vi "nanocal -- nuclear schottky fit V8.vi"() -> ()   [LabVIEW 2021] (continued)
0.000679567052   ,  \"σητN\" -> 0.003677742744    |>   , \r\"IDS0337_210904_RAW_cal__sam_\" ->   <|    \"ζ\" -> 0.174989526301   ,  \"τ1\" -> 0.032277116931   ,  \"τS\" -> 0.156061636315   ,  \"τN\" -> 0.033861256896   ,  \"τC\" -> 0.001461638306   ,  \"κ0\" -> 0.000000000742   ,  \"mm1\" -> 0.000216209109   ,  \"mm2\" -> 0.025810900049   ,  \"mm3\" -> 0.230869056407   ,  \"T\" -> 0.157000000000   ,  \"B\" -> 5.000000000000   ,  \"θ\" -> 90.000000000000   ,  \"Reoff\" -> -41753012.048192769300   ,  \"Imoff\" -> 0.000000000000   ,  \"στ1\" -> 0.000000000000   ,  \"στS\" -> 0.000000000000   ,  \"στN\" -> 0.000000000000   ,  \"τ11 \" -> 0.000000000000   ,  \"τ12\" -> 0.000000000000   ,  \"τ22\" -> 0.000000000000   ,  \"τN1\" -> 0.000000000000   ,  \"τN2\" -> 0.000000000000   ,  \"σηlogτ1 \" -> 0.000000000000   ,  \"σηlogτS\" -> 0.000000000000   ,  \"σηlogτN\" -> 0.000000000000   ,  \"σlogτ1\" -> 0.000000000000   ,  \"σlogτS\" -> 0.000000000000   ,  \"σlogτN\" -> 0.000000000000   ,  \"σητ1\" -> 0.000000000000   ,  \"σητS \" -> 0.000000000000   ,  \"σητN\" -> 0.000000000000    |>   , \r\"IDS0338_210904_RAW_cal__ref_\" ->   <|    \"ζ\" -> 0.265658527884   ,  \"τ1\" -> 0.023120075726   ,  \"τS\" -> 0.103313442466   ,  \"τN\" -> 0.020697464258   ,  \"τC\" -> 0.000912229768   ,  \"κ0\" -> 0.000000000737   ,  \"mm1\" -> 0.000190421822   ,  \"mm2\" -> 0.018760460104   ,  \"mm3\" -> 0.162036885215   ,  \"T\" -> 0.170000000000   ,  \"B\" -> 5.000000000000   ,  \"θ\" -> 90.000000000000   ,  \"Reoff\" -> 0.000000000000   ,  \"Imoff\" -> 0.000000000000   ,  \"στ1\" -> 0.000288316469   ,  \"στS\" -> 0.000137331811   ,  \"στN\" -> 0.000137381757   ,  \"τ11 \" -> 0.000000000000   ,  \"τ12\" -> 0.000000000000   ,  \"τ22\" -> 0.000000000000   ,  \"τN1\" -> 0.000000000000   ,  \"τN2\" -> 0.000000000000   ,  \"σηlogτ1 \" -> 0.284385432190   ,  \"σηlogτS\" -> 0.006339746651   ,  \"σηlogτN\" -> 0.161800590932   ,  \"σlogτ1\" -> 0.012470394664   ,  \"σlogτS\" -> 0.001329273401   ,  \"σlogτN\" -> 0.006637612960   ,  \"σητ1\" -> 0.006575012728   ,  \"σητS \" -> 0.000654981051   ,  \"σητN\" -> 0.003348861948    |>   , \r\"IDS0338_210904_RAW_cal__sam_\" ->   <|    \"ζ\" -> 0.165649151389   ,  \"τ1\" -> 0.028874600848   ,  \"τS\" -> 0.141983523605   ,  \"τN\" -> 0.021766467668   ,  \"τC\" -> 0.001383503895   ,  \"κ0\" -> 0.000000000838   ,  \"mm1\" -> 0.000195205233   ,  \"mm2\" -> 0.024502619119   ,  \"mm3\" -> 0.196435318758   ,  \"T\" -> 0.170000000000   ,  \"B\" -> 5.000000000000   ,  \"θ\" -> 90.000000000000   ,  \"Reoff\" -> -35397590.361445784600   ,  \"Imoff\" -> 0.000000000000   ,  \"στ1\" -> 0.000000000000   ,  \"στS\" -> 0.000000000000   ,  \"στN\" -> 0.000000000000   ,  \"τ11 \" -> 0.000000000000   ,  \"τ12\" -> 0.000000000000   ,  \"τ22\" -> 0.000000000000   ,  \"τN1\" -> 0.000000000000   ,  \"τN2\" -> 0.000000000000   ,  \"σηlogτ1 \" -> 0.000000000000   ,  \"σηlogτS\" -> 0.000000000000   ,  \"σηlogτN\" -> 0.000000000000   ,  \"σlogτ1\" -> 0.000000000000   ,  \"σlogτS\" -> 0.000000000000   ,  \"σlogτN\" -> 0.000000000000   ,  \"σητ1\" -> 0.000000000000   ,  \"σητS \" -> 0.000000000000   ,  \"σητN\" -> 0.000000000000    |>   , \r\"IDS0339_210904_RAW_cal__ref_\" ->   <|    \"ζ\" -> 0.114039542964   ,  \"τ1\" -> 0.023293546514   ,  \"τS\" -> 0.060135025475   ,  \"τN\" -> 0.005147326644   ,  \"τC\" -> 0.001354301187   ,  \"κ0\" -> 0.000000001349   ,  \"mm1\" -> 0.000136157097   ,  \"mm2\" -> 0.020781344891   ,  \"mm3\" -> 0.076457467431   ,  \"T\" -> 0.255000000000   ,  \"B\" -> 5.000000000000   ,  \"θ\" -> 90.000000000000   ,  \"Reoff\" -> 0.000000000000   ,  \"Imoff\" -> 0.000000000000   ,  \"στ1\" -> 0.000249233332   ,  \"στS\" -> 0.000026082358   ,  \"στN\" -> 0.000027486518   ,  \"τ11 \" -> 0.000000000000   ,  \"τ12\" -> 0.000000000000   ,  \"τ22\" -> 0.000000000000   ,  \"τN1\" -> 0.000000000000   ,  \"τN2\" -> 0.000000000000   ,  \"σηlogτ1 \" -> 0.202736508629   ,  \"σηlogτS\" -> 0.001489466713   ,  \"σηlogτN\" -> 0.146001002326   ,  \"σlogτ1\" -> 0.010699673046   ,  \"σlogτS\" -> 0.000433729889   ,  \"σlogτN\" -> 0.005339959858   ,  \"σητ1\" -> 0.004722452294   ,  \"σητS \" -> 0.000089569119   ,  \"σητN\" -> 0.000751514849    |>   , \r\"IDS0339_210904_RAW_cal__sam_\" ->   <|    \"ζ\" -> 0.070510248751   ,  \"τ1\" -> 0.022152847239   ,  \"τS\" -> 0.078660981887   ,  \"τN\" -> 0.006346817462   ,  \"τC\" -> 0.001852903257   ,  \"κ0\" -> 0.000000001477   ,  \"mm1\" -> 0.000119580835   ,  \"mm2\" -> 0.020081415868   ,  \"mm3\" -> 0.094806474219   ,  \"T\" -> 0.255000000000   ,  \"B\" -> 5.000000000000   ,  \"θ\" -> 90.000000000000   ,  \"Reoff\" -> -9000000.000000000000   ,  \"Imoff\" -> 0.000000000000   ,  \"στ1\" -> 0.000000000000   ,  \"στS\" -> 0.000000000000   ,  \"στN\" -> 0.000000000000   ,  \"τ11 \" -> 0.000000000000   ,  \"τ12\" -> 0.000000000000   ,  \"τ22\" -> 0.000000000000   ,  \"τN1\" -> 0.000000000000   ,  \"τN2\" -> 0.000000000000   ,  \"σηlogτ1 \" -> 0.000000000000   ,  \"σηlogτS\" -> 0.000000000000   ,  \"σηlogτN\" -> 0.000000000000   ,  \"σlogτ1\" -> 0.000000000000   ,  \"σlogτS\" -> 0.000000000000   ,  \"σlogτN\" -> 0.000000000000   ,  \"σητ1\" -> 0.000000000000   ,  \"σητS \" -> 0.000000000000   ,  \"σητN\" -> 0.000000000000    |>   , \r\"IDS0340_210904_RAW_cal__ref_\" ->   <|    \"ζ\" -> 0.076525648542   ,  \"τ1\" -> 0.027695674574   ,  \"τS\" -> 0.050135533571   ,  \"τN\" -> 0.002521537223   ,  \"τC\" -> 0.001686073318   ,  \"κ0\" -> 0.000000001730   ,  \"mm1\" -> 0.000116467999   ,  \"mm2\" -> 0.025407303981   ,  \"mm3\" -> 0.060544663199   ,  \"T\" -> 0.308000000000   ,  \"B\" -> 5.000000000000   ,  \"θ\" -> 90.000000000000   ,  \"Reoff\" -> 0.000000000000   ,  \"Imoff\" -> 0.000000000000   ,  \"στ1\" -> 0.000231753766   ,  \"στS\" -> 0.000008787417   ,  \"στN\" -> 0.000010480438   ,  \"τ11 \" -> 0.000000000000   ,  \"τ12\" -> 0.000000000000   ,  \"τ22\" -> 0.000000000000   ,  \"τN1\" -> 0.000000000000   ,  \"τN2\" -> 0.000000000000   ,  \"σηlogτ1 \" -> 0.162472207290   ,  \"σηlogτS\" -> 0.000540904127   ,  \"σηlogτN\" -> 0.139012219140   ,  \"σlogτ1\" -> 0.008367868614   ,  \"σlogτS\" -> 0.000175273227   ,  \"σlogτN\" -> 0.004156368718   ,  \"σητ1\" -> 0.004499777380   ,  \"σητS \" -> 0.000027118517   ,  \"σητN\" -> 0.000350524485    |>   , \r\"IDS0340_210904_RAW_cal__sam_\" ->   <|    \"ζ\" -> 0.049192434897   ,  \"τ1\" -> 0.021139048522   ,  \"τS\" -> 0.064524263818   ,  \"τN\" -> 0.003413094239   ,  \"τC\" -> 0.002227810965   ,  \"κ0\" -> 0.000000001879   ,  \"mm1\" -> 0.000101271202   ,  \"mm2\" -> 0.019728994700   ,  \"mm3\" -> 0.074815955705   ,  \"T\" -> 0.308000000000   ,  \"B\" -> 5.000000000000   ,  \"θ\" -> 90.000000000000   ,  \"Reoff\" -> -4933734.939759036530   ,  \"Imoff\" -> 0.000000000000   ,  \"στ1\" -> 0.000000000000   ,  \"στS\" -> 0.000000000000   ,  \"στN\" -> 0.000000000000   ,  \"τ11 \" -> 0.000000000000   ,  \"τ12\" -> 0.000000000000   ,  \"τ22\" -> 0.000000000000   ,  \"τN1\" -> 0.000000000000   ,  \"τN2\" -> 0.000000000000   ,  \"σηlogτ1 \" -> 0.000000000000   ,  \"σηlogτS\" -> 0.000000000000   ,  \"σηlogτN\" -> 0.000000000000   ,  \"σlogτ1\" -> 0.000000000000   ,  \"σlogτS\" -> 0.000000000000   ,  \"σlogτN\" -> 0.000000000000   ,  \"σητ1\" -> 0.000000000000   ,  \"σητS \" -> 0.000000000000   ,  \"σητN\" -> 0.000000000000    |>   , \r\"IDS0341_210904_RAW_cal__ref_\" ->   <|    \"ζ\" -> 0.056782811482   ,  \"τ1\" -> 0.026331968848   ,  \"τS\" -> 0.042767805397   ,  \"τN\" -> 0.001889396139   ,  \"τC\" -> 0.002016272015   ,  \"κ0\" -> 0.000000002097   ,  \"mm1\" -> 0.000103939246   ,  \"mm2\" -> 0.024219601276   ,  \"mm3\" -> 0.051217663333   ,  \"T\" -> 0.360000000000   ,  \"B\" -> 5.000000000000   ,  \"θ\" -> 90.000000000000   ,  \"Reoff\" -> 0.000000000000   ,  \"Imoff\" -> 0.000000000000   ,  \"στ1\" -> 0.000101422442   ,  \"στS\" -> 0.000002887305   ,  \"στN\" -> 0.000003653210   ,  \"τ11 \" -> 0.000000000000   ,  \"τ12\" -> 0.000000000000   ,  \"τ22\" -> 0.000000000000   ,  \"τN1\" -> 0.000000000000   ,  \"τN2\" -> 0.000000000000   ,  \"σηlogτ1 \" -> 0.151982642430   ,  \"σηlogτS\" -> 0.000404656843   ,  \"σηlogτN\" -> 0.137111244570   ,  \"σlogτ1\" -> 0.003851684700   ,  \"σlogτS\" -> 0.000067511173   ,  \"σlogτN\" -> 0.001933533055   ,  \"σητ1\" -> 0.004002002206   ,  \"σητS \" -> 0.000017306285   ,  \"σητN\" -> 0.000259057456    |>   , \r\"IDS0341_210904_RAW_cal__sam_\" ->   <|    \"ζ\" -> 0.036062522071   ,  \"τ1\" -> 0.018116162768   ,  \"τS\" -> 0.055032833309   ,  \"τN\" -> 0.002026723445   ,  \"τC\" -> 0.002755523522   ,  \"κ0\" -> 0.000000002282   ,  \"mm1\" -> 0.000091630452   ,  \"mm2\" -> 0.017261892165   ,  \"mm3\" -> 0.062635431951   ,  \"T\" -> 0.360000000000   ,  \"B\" -> 5.000000000000   ,  \"θ\" -> 90.000000000000   ,  \"Reoff\" -> -2587349.397590361540   ,  \"Imoff\" -> 0.000000000000   ,  \"στ1\" -> 0.000000000000   ,  \"στS\" -> 0.000000000000   ,  \"στN\" -> 0.000000000000   ,  \"τ11 \" -> 0.000000000000   ,  \"τ12\" -> 0.000000000000   ,  \"τ22\" -> 0.000000000000   ,  \"τN1\" -> 0.000000000000   ,  \"τN2\" -> 0.000000000000   ,  \"σηlogτ1 \" -> 0.000000000000   ,  \"σηlogτS\" -> 0.000000000000   ,  \"σηlogτN\" -> 0.000000000000   ,  \"σlogτ1\" -> 0.000000000000   ,  \"σlogτS\" -> 0.000000000000   ,  \"σlogτN\" -> 0.000000000000   ,  \"σητ1\" -> 0.000000000000   ,  \"σητS \" -> 0.000000000000   ,  \"σητN\" -> 0.000000000000    |>   , \r\"IDS0342_210904_RAW_cal__ref_\" ->   <|    \"ζ\" -> 0.041076601022   ,  \"τ1\" -> 0.018757031155   ,  \"τS\" -> 0.035968750366   ,  \"τN\" -> 0.001085416882   ,  \"τC\" -> 0.002380872433   ,  \"κ0\" -> 0.000000002638   ,  \"mm1\" -> 0.000088519730   ,  \"mm2\" -> 0.017837018320   ,  \"mm3\" -> 0.041788592031   ,  \"T\" -> 0.438000000000   ,  \"B\" -> 5.000000000000   ,  \"θ\" -> 90.000000000000   ,  \"Reoff\" -> 0.000000000000   ,  \"Imoff\" -> 0.000000000000   ,  \"στ1\" -> 0.000064198355   ,  \"στS\" -> 0.000001597078   ,  \"στN\" -> 0.000001834209   ,  \"τ11 \" -> 0.000000000000   ,  \"τ12\" -> 0.000000000000   ,  \"τ22\" -> 0.000000000000   ,  \"τN1\" -> 0.000000000000   ,  \"τN2\" -> 0.000000000000   ,  \"σηlogτ1 \" -> 0.168171879856   ,  \"σηlogτS\" -> 0.000355670898   ,  \"σηlogτN\" -> 0.139592379603   ,  \"σlogτ1\" -> 0.003422628813   ,  \"σlogτS\" -> 0.000044401831   ,  \"σlogτN\" -> 0.001689865537   ,  \"σητ1\" -> 0.003154405190   ,  \"σητS \" -> 0.000012793038   ,  \"σητN\" -> 0.000151515925    |>   , \r\"IDS0342_210904_RAW_cal__sam_\" ->   <|    \"ζ\" -> 0.027534849374   ,  \"τ1\" -> 0.019066527741   ,  \"τS\" -> 0.046236587360   ,  \"τN\" -> 0.001227722560   ,  \"τC\" -> 0.003332461518   ,  \"κ0\" -> 0.000000002852   ,  \"mm1\" -> 0.000083583563   ,  \"mm2\" -> 0.018352322518   ,  \"mm3\" -> 0.052734315722   ,  \"T\" -> 0.438000000000   ,  \"B\" -> 5.000000000000   ,  \"θ\" -> 90.000000000000   ,  \"Reoff\" -> -1846385.542168676850   ,  \"Imoff\" -> 0.000000000000   ,  \"στ1\" -> 0.000000000000   ,  \"στS\" -> 0.000000000000   ,  \"στN\" -> 0.000000000000   ,  \"τ11 \" -> 0.000000000000   ,  \"τ12\" -> 0.000000000000   ,  \"τ22\" -> 0.000000000000   ,  \"τN1\" -> 0.000000000000   ,  \"τN2\" -> 0.000000000000   ,  \"σηlogτ1 \" -> 0.000000000000   ,  \"σηlogτS\" -> 0.000000000000   ,  \"σηlogτN\" -> 0.000000000000   ,  \"σlogτ1\" -> 0.000000000000   ,  \"σlogτS\" -> 0.000000000000   ,  \"σlogτN\" -> 0.000000000000   ,  \"σητ1\" -> 0.000000000000   ,  \"σητS \" -> 0.000000000000   ,  \"σητN\" -> 0.000000000000    |>   , \r\"IDS0343_210904_RAW_cal__ref_\" ->   <|    \"ζ\" -> 0.030668897536   ,  \"τ1\" -> 0.016422384876   ,  \"τS\" -> 0.030525750501   ,  \"τN\" -> 0.000737103869   ,  \"τC\" -> 0.002827601045   ,  \"κ0\" -> 0.000000003285   ,  \"mm1\" -> 0.000077374536   ,  \"mm2\" -> 0.015772817310   ,  \"mm3\" -> 0.035621445722   ,  \"T\" -> 0.530000000000   ,  \"B\" -> 5.000000000000   ,  \"θ\" -> 90.000000000000   ,  \"Reoff\" -> 0.000000000000   ,  \"Imoff\" -> 0.000000000000   ,  \"στ1\" -> 0.000085303275   ,  \"στS\" -> 0.000001638656   ,  \"στN\" -> 0.000001890230   ,  \"τ11 \" -> 0.000000000000   ,  \"τ12\" -> 0.000000000000   ,  \"τ22\" -> 0.000000000000   ,  \"τN1\" -> 0.000000000000   ,  \"τN2\" -> 0.000000000000   ,  \"σηlogτ1 \" -> 0.166582880232   ,  \"σηlogτS\" -> 0.000279115337   ,  \"σηlogτN\" -> 0.139234460334   ,  \"σlogτ1\" -> 0.005194329317   ,  \"σlogτS\" -> 0.000053681095   ,  \"σlogτN\" -> 0.002564401366   ,  \"σητ1\" -> 0.002735688173   ,  \"σητS \" -> 0.000008520205   ,  \"σητN\" -> 0.000102630259    |>   , \r\"IDS0343_210904_RAW_cal__sam_\" ->   <|    \"ζ\" -> 0.023098882919   ,  \"τ1\" -> 0.017709986922   ,  \"τS\" -> 0.038881575014   ,  \"τN\" -> 0.000747654909   ,  \"τC\" -> 0.003803962289   ,  \"κ0\" -> 0.000000003538   ,  \"mm1\" -> 0.000078528513   ,  \"mm2\" -> 0.017209583260   ,  \"mm3\" -> 0.044770458303   ,  \"T\" -> 0.530000000000   ,  \"B\" -> 5.000000000000   ,  \"θ\" -> 90.000000000000   ,  \"Reoff\" -> -1599397.590361446140   ,  \"Imoff\" -> 0.000000000000   ,  \"στ1\" -> 0.000000000000   ,  \"στS\" -> 0.000000000000   ,  \"στN\" -> 0.000000000000   ,  \"τ11 \" -> 0.000000000000   ,  \"τ12\" -> 0.000000000000   ,  \"τ22\" -> 0.000000000000   ,  \"τN1\" -> 0.000000000000   ,  \"τN2\" -> 0.000000000000   ,  \"σηlogτ1 \" -> 0.000000000000   ,  \"σηlogτS\" -> 0.000000000000   ,  \"σηlogτN\" -> 0.000000000000   ,  \"σlogτ1\" -> 0.000000000000   ,  \"σlogτS\" -> 0.000000000000   ,  \"σlogτN\" -> 0.000000000000   ,  \"σητ1\" -> 0.000000000000   ,  \"σητS \" -> 0.000000000000   ,  \"σητN\" -> 0.000000000000    |>   , \r\"IDS0344_210904_RAW_cal__ref_\" ->   <|    \"ζ\" -> 0.026709812446   ,  \"τ1\" -> 0.026755113102   ,  \"τS\" -> 0.027056221253   ,  \"τN\" -> 0.000433685724   ,  \"τC\" -> 0.002938863970   ,  \"κ0\" -> 0.000000003892   ,  \"mm1\" -> 0.000069295841   ,  \"mm2\" -> 0.024848155483   ,  \"mm3\" -> 0.033000682984   ,  \"T\" -> 0.620000000000   ,  \"B\" -> 5.000000000000   ,  \"θ\" -> 90.000000000000   ,  \"Reoff\" -> 0.000000000000   ,  \"Imoff\" -> 0.000000000000   ,  \"στ1\" -> 0.000318098856   ,  \"στS\" -> 0.000001623783   ,  \"στN\" -> 0.000002850113   ,  \"τ11 \" -> 0.000000000000   ,  \"τ12\" -> 0.000000000000   ,  \"τ22\" -> 0.000000000000   ,  \"τN1\" -> 0.000000000000   ,  \"τN2\" -> 0.000000000000   ,  \"σηlogτ1 \" -> 0.118559715842   ,  \"σηlogτS\" -> 0.000074397800   ,  \"σηlogτN\" -> 0.130425012097   ,  \"σlogτ1\" -> 0.011889273453   ,  \"σlogτS\" -> 0.000060015159   ,  \"σlogτN\" -> 0.006571839401   ,  \"σητ1\" -> 0.003172078607   ,  \"σητS \" -> 0.000002012923   ,  \"σητN\" -> 0.000056563466    |>   , \r\"IDS0344_210904_RAW_cal__sam_\" ->   <|    \"ζ\" -> 0.019239644947   ,  \"τ1\" -> 0.016162010817   ,  \"τS\" -> 0.033688234899   ,  \"τN\" -> 0.000426792406   ,  \"τC\" -> 0.004393456024   ,  \"κ0\" -> 0.000000004224   ,  \"mm1\" -> 0.000073664779   ,  \"mm2\" -> 0.015859557336   ,  \"mm3\" -> 0.039393633044   ,  \"T\" -> 0.620000000000   ,  \"B\" -> 5.000000000000   ,  \"θ\" -> 90.000000000000   ,  \"Reoff\" -> -1105421.686746988450   ,  \"Imoff\" -> 0.000000000000   ,  \"στ1\" -> 0.000000000000   ,  \"στS\" -> 0.000000000000   ,  \"στN\" -> 0.000000000000   ,  \"τ11 \" -> 0.000000000000   ,  \"τ12\" -> 0.000000000000   ,  \"τ22\" -> 0.000000000000   ,  \"τN1\" -> 0.000000000000   ,  \"τN2\" -> 0.000000000000   ,  \"σηlogτ1 \" -> 0.000000000000   ,  \"σηlogτS\" -> 0.000000000000   ,  \"σηlogτN\" -> 0.000000000000   ,  \"σlogτ1\" -> 0.000000000000   ,  \"σlogτS\" -> 0.000000000000   ,  \"σlogτN\" -> 0.000000000000   ,  \"σητ1\" -> 0.000000000000   ,  \"σητS \" -> 0.000000000000   ,  \"σητN\" -> 0.000000000000    |>   , \r\"IDS0346_210904_RAW_cal__ref_\" ->   <|    \"ζ\" -> 0.407818389237   ,  \"τ1\" -> 0.059098367304   ,  \"τS\" -> 0.136395388136   ,  \"τN\" -> 0.197758233370   ,  \"τC\" -> 0.001024329886   ,  \"κ0\" -> 0.000000000393   ,  \"mm1\" -> 0.000295598957   ,  \"mm2\" -> 0.022431935370   ,  \"mm3\" -> 0.507822776049   ,  \"T\" -> 0.122000000000   ,  \"B\" -> 8.000000000000   ,  \"θ\" -> 90.000000000000   ,  \"Reoff\" -> 0.000000000000   ,  \"Imoff\" -> 0.000000000000   ,  \"στ1\" -> 0.000493664169   ,  \"στS\" -> 0.000493598095   ,  \"στN\" -> 0.000812310097   ,  \"τ11 \" -> 0.000000000000   ,  \"τ12\" -> 0.000000000000   ,  \"τ22\" -> 0.000000000000   ,  \"τN1\" -> 0.000000000000   ,  \"τN2\" -> 0.000000000000   ,  \"σηlogτ1 \" -> 0.194694000050   ,  \"σηlogτS\" -> 0.012711324010   ,  \"σηlogτN\" -> 0.173317416285   ,  \"σlogτ1\" -> 0.008353262390   ,  \"σlogτS\" -> 0.003618876720   ,  \"σlogτN\" -> 0.004107591797   ,  \"σητ1\" -> 0.011506097527   ,  \"σητS \" -> 0.001733765972   ,  \"σητN\" -> 0.034274946057    |>   , \r\"IDS0346_210904_RAW_cal__sam_\" ->   <|    \"ζ\" -> 0.199267253863   ,  \"τ1\" -> 0.050205114691   ,  \"τS\" -> 0.125855812683   ,  \"τN\" -> 0.296749666016   ,  \"τC\" -> 0.001624351903   ,  \"κ0\" -> 0.000000000535   ,  \"mm1\" -> 0.000267463038   ,  \"mm2\" -> 0.014047868056   ,  \"mm3\" -> 0.544331047407   ,  \"T\" -> 0.122000000000   ,  \"B\" -> 8.000000000000   ,  \"θ\" -> 90.000000000000   ,  \"Reoff\" -> -35716867.469879508000   ,  \"Imoff\" -> 0.000000000000   ,  \"στ1\" -> 0.000000000000   ,  \"στS\" -> 0.000000000000   ,  \"στN\" -> 0.000000000000   ,  \"τ11 \" -> 0.000000000000   ,  \"τ12\" -> 0.000000000000   ,  \"τ22\" -> 0.000000000000   ,  \"τN1\" -> 0.000000000000   ,  \"τN2\" -> 0.000000000000   ,  \"σηlogτ1 \" -> 0.000000000000   ,  \"σηlogτS\" -> 0.000000000000   ,  \"σηlogτN\" -> 0.000000000000   ,  \"σlogτ1\" -> 0.000000000000   ,  \"σlogτS\" -> 0.000000000000   ,  \"σlogτN\" -> 0.000000000000   ,  \"σητ1\" -> 0.000000000000   ,  \"σητS \" -> 0.000000000000   ,  \"σητN\" -> 0.000000000000    |>   , \r\"IDS0347_210906_RAW_cal__ref_\" ->   <|    \"ζ\" -> 0.290481808635   ,  \"τ1\" -> 0.038323944120   ,  \"τS\" -> 0.067047611498   ,  \"τN\" -> 0.095881318046   ,  \"τC\" -> 0.000911015117   ,  \"κ0\" -> 0.000000000644   ,  \"mm1\" -> 0.000203389328   ,  \"mm2\" -> 0.014222650453   ,  \"mm3\" -> 0.235065739133   ,  \"T\" -> 0.157000000000   ,  \"B\" -> 8.000000000000   ,  \"θ\" -> 90.000000000000   ,  \"Reoff\" -> 0.000000000000   ,  \"Imoff\" -> 0.000000000000   ,  \"στ1\" -> 0.000081642608   ,  \"στS\" -> 0.000055996925   ,  \"στN\" -> 0.000108329720   ,  \"τ11 \" -> 0.000000000000   ,  \"τ12\" -> 0.000000000000   ,  \"τ22\" -> 0.000000000000   ,  \"τN1\" -> 0.000000000000   ,  \"τN2\" -> 0.000000000000   ,  \"σηlogτ1 \" -> 0.166799167293   ,  \"σηlogτS\" -> 0.009320651053   ,  \"σηlogτN\" -> 0.160780135489   ,  \"σlogτ1\" -> 0.002130328947   ,  \"σlogτS\" -> 0.000835181511   ,  \"σlogτN\" -> 0.001129831357   ,  \"σητ1\" -> 0.006392401967   ,  \"σητS \" -> 0.000624927391   ,  \"σητN\" -> 0.015415811306    |>   , \r\"IDS0347_210906_RAW_cal__sam_\" ->   <|    \"ζ\" -> 0.169709128246   ,  \"τ1\" -> 0.042569783210   ,  \"τS\" -> 0.096466158196   ,  \"τN\" -> 0.116379310482   ,  \"τC\" -> 0.001498996005   ,  \"κ0\" -> 0.000000000766   ,  \"mm1\" -> 0.000215022431   ,  \"mm2\" -> 0.017656553883   ,  \"mm3\" -> 0.275164490520   ,  \"T\" -> 0.157000000000   ,  \"B\" -> 8.000000000000   ,  \"θ\" -> 90.000000000000   ,  \"Reoff\" -> -35716867.469879508000   ,  \"Imoff\" -> 0.000000000000   ,  \"στ1\" -> 0.000000000000   ,  \"στS\" -> 0.000000000000   ,  \"στN\" -> 0.000000000000   ,  \"τ11 \" -> 0.000000000000   ,  \"τ12\" -> 0.000000000000   ,  \"τ22\" -> 0.000000000000   ,  \"τN1\" -> 0.000000000000   ,  \"τN2\" -> 0.000000000000   ,  \"σηlogτ1 \" -> 0.000000000000   ,  \"σηlogτS\" -> 0.000000000000   ,  \"σηlogτN\" -> 0.000000000000   ,  \"σlogτ1\" -> 0.000000000000   ,  \"σlogτS\" -> 0.000000000000   ,  \"σlogτN\" -> 0.000000000000   ,  \"σητ1\" -> 0.000000000000   ,  \"σητS \" -> 0.000000000000   ,  \"σητN\" -> 0.000000000000    |>   , \r\"IDS0348_210906_RAW_cal__ref_\" ->   <|    \"ζ\" -> 0.234564712181   ,  \"τ1\" -> 0.031261792512   ,  \"τS\" -> 0.052786157224   ,  \"τN\" -> 0.062944714793   ,  \"τC\" -> 0.000875309632   ,  \"κ0\" -> 0.000000000764   ,  \"mm1\" -> 0.000164501338   ,  \"mm2\" -> 0.012702176672   ,  \"mm3\" -> 0.162147674837   ,  \"T\" -> 0.178000000000   ,  \"B\" -> 8.000000000000   ,  \"θ\" -> 90.000000000000   ,  \"Reoff\" -> 0.000000000000   ,  \"Imoff\" -> 0.000000000000   ,  \"στ1\" -> 0.000050446338   ,  \"στS\" -> 0.000029155358   ,  \"στN\" -> 0.000054402622   ,  \"τ11 \" -> 0.000000000000   ,  \"τ12\" -> 0.000000000000   ,  \"τ22\" -> 0.000000000000   ,  \"τN1\" -> 0.000000000000   ,  \"τN2\" -> 0.000000000000   ,  \"σηlogτ1 \" -> 0.161173739457   ,  \"σηlogτS\" -> 0.007924149958   ,  \"σηlogτN\" -> 0.155365649649   ,  \"σlogτ1\" -> 0.001613673870   ,  \"σlogτS\" -> 0.000552329615   ,  \"σlogτN\" -> 0.000864292135   ,  \"σητ1\" -> 0.005038580001   ,  \"σητS \" -> 0.000418285426   ,  \"σητN\" -> 0.009779446506    |>   , \r\"IDS0348_210906_RAW_cal__sam_\" ->   <|    \"ζ\" -> 0.135783247929   ,  \"τ1\" -> 0.037121050091   ,  \"τS\" -> 0.079201640502   ,  \"τN\" -> 0.079201640502   ,  \"τC\" -> 0.001474311209   ,  \"κ0\" -> 0.000000000894   ,  \"mm1\" -> 0.000173730712   ,  \"mm2\" -> 0.016810842330   ,  \"mm3\" -> 0.201522581240   ,  \"T\" -> 0.178000000000   ,  \"B\" -> 8.000000000000   ,  \"θ\" -> 90.000000000000   ,  \"Reoff\" -> -29680722.891566276600   ,  \"Imoff\" -> 0.000000000000   ,  \"στ1\" -> 0.000000000000   ,  \"στS\" -> 0.000000000000   ,  \"στN\" -> 0.000000000000   ,  \"τ11 \" -> 0.000000000000   ,  \"τ12\" -> 0.000000000000   ,  \"τ22\" -> 0.000000000000   ,  \"τN1\" -> 0.000000000000   ,  \"τN2\" -> 0.000000000000   ,  \"σηlogτ1 \" -> 0.000000000000   ,  \"σηlogτS\" -> 0.000000000000   ,  \"σηlogτN\" -> 0.000000000000   ,  \"σlogτ1\" -> 0.000000000000   ,  \"σlogτS\" -> 0.000000000000   ,  \"σlogτN\" -> 0.000000000000   ,  \"σητ1\" -> 0.000000000000   ,  \"σητS \" -> 0.000000000000   ,  \"σητN\" -> 0.000000000000    |>   , \r\"IDS0349_210906_RAW_cal__ref_\" ->   <|    \"ζ\" -> 0.197057469427   ,  \"τ1\" -> 0.029613620558   ,  \"τS\" -> 0.050911815815   ,  \"τN\" -> 0.036816442025   ,  \"τC\" -> 0.000965034060   ,  \"κ0\" -> 0.000000001032   ,  \"mm1\" -> 0.000156774968   ,  \"mm2\" -> 0.015211417778   ,  \"mm3\" -> 0.120226228199   ,  \"T\" -> 0.200000000000   ,  \"B\" -> 8.000000000000   ,  \"θ\" -> 90.000000000000   ,  \"Reoff\" -> 0.000000000000   ,  \"Imoff\" -> 0.000000000000   ,  \"στ1\" -> 0.000057169127   ,  \"στS\" -> 0.000023609008   ,  \"στN\" -> 0.000037318979   ,  \"τ11 \" -> 0.000000000000   ,  \"τ12\" -> 0.000000000000   ,  \"τ22\" -> 0.000000000000   ,  \"τN1\" -> 0.000000000000   ,  \"τN2\" -> 0.000000000000   ,  \"σηlogτ1 \" -> 0.161376688793   ,  \"σηlogτS\" -> 0.005816962816   ,  \"σηlogτN\" -> 0.148995950079   ,  \"σlogτ1\" -> 0.001930501090   ,  \"σlogτS\" -> 0.000463723546   ,  \"σlogτN\" -> 0.001013649805   ,  \"σητ1\" -> 0.004778948029   ,  \"σητS \" -> 0.000296152139   ,  \"σητN\" -> 0.005485500758    |>   , \r\"IDS0349_210906_RAW_cal__sam_\" ->   <|    \"ζ\" -> 0.113690190882   ,  \"τ1\" -> 0.032691214581   ,  \"τS\" -> 0.068786957350   ,  \"τN\" -> 0.048058332081   ,  \"τC\" -> 0.001613875480   ,  \"κ0\" -> 0.000000001156   ,  \"mm1\" -> 0.000161675745   ,  \"mm2\" -> 0.017372504664   ,  \"mm3\" -> 0.146900362342   ,  \"T\" -> 0.200000000000   ,  \"B\" -> 8.000000000000   ,  \"θ\" -> 90.000000000000   ,  \"Reoff\" -> -14590361.445783138300   ,  \"Imoff\" -> 0.000000000000   ,  \"στ1\" -> 0.000000000000   ,  \"στS\" -> 0.000000000000   ,  \"στN\" -> 0.000000000000   ,  \"τ11 \" -> 0.000000000000   ,  \"τ12\" -> 0.000000000000   ,  \"τ22\" -> 0.000000000000   ,  \"τN1\" -> 0.000000000000   ,  \"τN2\" -> 0.000000000000   ,  \"σηlogτ1 \" -> 0.000000000000   ,  \"σηlogτS\" -> 0.000000000000   ,  \"σηlogτN\" -> 0.000000000000   ,  \"σlogτ1\" -> 0.000000000000   ,  \"σlogτS\" -> 0.000000000000   ,  \"σlogτN\" -> 0.000000000000   ,  \"σητ1\" -> 0.000000000000   ,  \"σητS \" -> 0.000000000000   ,  \"σητN\" -> 0.000000000000    |>   , \r\"IDS0350_210906_RAW_cal__ref_\" ->   <|    \"ζ\" -> 0.116383968065   ,  \"τ1\" -> 0.022837025685   ,  \"τS\" -> 0.041355624864   ,  \"τN\" -> 0.016243225582   ,  \"τC\" -> 0.001144746242   ,  \"κ0\" -> 0.000000001355   ,  \"mm1\" -> 0.000116736213   ,  \"mm2\" -> 0.014664448269   ,  \"mm3\" -> 0.073503020662   ,  \"T\" -> 0.260000000000   ,  \"B\" -> 8.000000000000   ,  \"θ\" -> 90.000000000000   ,  \"Reoff\" -> 0.000000000000   ,  \"Imoff\" -> 0.000000000000   ,  \"στ1\" -> 0.000027906584   ,  \"στS\" -> 0.000007380086   ,  \"στN\" -> 0.000010191855   ,  \"τ11 \" -> 0.000000000000   ,  \"τ12\" -> 0.000000000000   ,  \"τ22\" -> 0.000000000000   ,  \"τN1\" -> 0.000000000000   ,  \"τN2\" -> 0.000000000000   ,  \"σηlogτ1 \" -> 0.162256483080   ,  \"σηlogτS\" -> 0.003668520899   ,  \"σηlogτN\" -> 0.144232966841   ,  \"σlogτ1\" -> 0.001221988557   ,  \"σlogτS\" -> 0.000178454219   ,  \"σlogτN\" -> 0.000627452654   ,  \"σητ1\" -> 0.003705455472   ,  \"σητS \" -> 0.000151713974   ,  \"σητN\" -> 0.002342808617    |>   , \r\"IDS0350_210906_RAW_cal__sam_\" ->   <|    \"ζ\" -> 0.071614468485   ,  \"τ1\" -> 0.024327525692   ,  \"τS\" -> 0.055056024171   ,  \"τN\" -> 0.019709093999   ,  \"τC\" -> 0.001754398678   ,  \"κ0\" -> 0.000000001497   ,  \"mm1\" -> 0.000114067222   ,  \"mm2\" -> 0.016460052715   ,  \"mm3\" -> 0.089627186802   ,  \"T\" -> 0.260000000000   ,  \"B\" -> 8.000000000000   ,  \"θ\" -> 90.000000000000   ,  \"Reoff\" -> -10063253.012048184900   ,  \"Imoff\" -> 0.000000000000   ,  \"στ1\" -> 0.000000000000   ,  \"στS\" -> 0.000000000000   ,  \"στN\" -> 0.000000000000   ,  \"τ11 \" -> 0.000000000000   ,  \"τ12\" -> 0.000000000000   ,  \"τ22\" -> 0.000000000000   ,  \"τN1\" -> 0.000000000000   ,  \"τN2\" -> 0.000000000000   ,  \"σηlogτ1 \" -> 0.000000000000   ,  \"σηlogτS\" -> 0.000000000000   ,  \"σηlogτN\" -> 0.000000000000   ,  \"σlogτ1\" -> 0.000000000000   ,  \"σlogτS\" -> 0.000000000000   ,  \"σlogτN\" -> 0.000000000000   ,  \"σητ1\" -> 0.000000000000   ,  \"σητS \" -> 0.000000000000   ,  \"σητN\" -> 0.000000000000    |>   , \r\"IDS0351_210906_RAW_cal__ref_\" ->   <|    \"ζ\" -> 0.080064937947   ,  \"τ1\" -> 0.017296327437   ,  \"τS\" -> 0.036479707086   ,  \"τN\" -> 0.008116806938   ,  \"τC\" -> 0.001346314476   ,  \"κ0\" -> 0.000000001766   ,  \"mm1\" -> 0.000096730306   ,  \"mm2\" -> 0.013119572667   ,  \"mm3\" -> 0.053593470093   ,  \"T\" -> 0.310000000000   ,  \"B\" -> 8.000000000000   ,  \"θ\" -> 90.000000000000   ,  \"Reoff\" -> 0.000000000000   ,  \"Imoff\" -> 0.000000000000   ,  \"στ1\" -> 0.000031102743   ,  \"στS\" -> 0.000006077841   ,  \"στN\" -> 0.000007305969   ,  \"τ11 \" -> 0.000000000000   ,  \"τ12\" -> 0.000000000000   ,  \"τ22\" -> 0.000000000000   ,  \"τN1\" -> 0.000000000000   ,  \"τN2\" -> 0.000000000000   ,  \"σηlogτ1 \" -> 0.176104217691   ,  \"σηlogτS\" -> 0.002693810692   ,  \"σηlogτN\" -> 0.144358868609   ,  \"σlogτ1\" -> 0.001798228177   ,  \"σlogτS\" -> 0.000166608817   ,  \"σlogτN\" -> 0.000900103833   ,  \"σητ1\" -> 0.003045956212   ,  \"σητS \" -> 0.000098269425   ,  \"σητN\" -> 0.001171733066    |>   , \r\"IDS0351_210906_RAW_cal__sam_\" ->   <|    \"ζ\" -> 0.049866383839   ,  \"τ1\" -> 0.023285662985   ,  \"τS\" -> 0.049370833464   ,  \"τN\" -> 0.009866658615   ,  \"τC\" -> 0.002153040267   ,  \"κ0\" -> 0.000000001928   ,  \"mm1\" -> 0.000098362318   ,  \"mm2\" -> 0.018063601956   ,  \"mm3\" -> 0.069468190575   ,  \"T\" -> 0.310000000000   ,  \"B\" -> 8.000000000000   ,  \"θ\" -> 90.000000000000   ,  \"Reoff\" -> -5536144.578313261270   ,  \"Imoff\" -> 0.000000000000   ,  \"στ1\" -> 0.000000000000   ,  \"στS\" -> 0.000000000000   ,  \"στN\" -> 0.000000000000   ,  \"τ11 \" -> 0.000000000000   ,  \"τ12\" -> 0.000000000000   ,  \"τ22\" -> 0.000000000000   ,  \"τN1\" -> 0.000000000000   ,  \"τN2\" -> 0.000000000000   ,  \"σηlogτ1 \" -> 0.000000000000   ,  \"σηlogτS\" -> 0.000000000000   ,  \"σηlogτN\" -> 0.000000000000   ,  \"σlogτ1\" -> 0.000000000000   ,  \"σlogτS\" -> 0.000000000000   ,  \"σlogτN\" -> 0.000000000000   ,  \"σητ1\" -> 0.000000000000   ,  \"σητS \" -> 0.000000000000   ,  \"σητN\" -> 0.000000000000    |>   , \r\"IDS0352_210906_RAW_cal__ref_\" ->   <|    \"ζ\" -> 0.060178216595   ,  \"τ1\" -> 0.015538327560   ,  \"τS\" -> 0.033922393417   ,  \"τN\" -> 0.005018769313   ,  \"τC\" -> 0.001649636137   ,  \"κ0\" -> 0.000000002110   ,  \"mm1\" -> 0.000089741441   ,  \"mm2\" -> 0.012788298805   ,  \"mm3\" -> 0.045594495906   ,  \"T\" -> 0.360000000000   ,  \"B\" -> 8.000000000000   ,  \"θ\" -> 90.000000000000   ,  \"Reoff\" -> 0.000000000000   ,  \"Imoff\" -> 0.000000000000   ,  \"στ1\" -> 0.000024762200   ,  \"στS\" -> 0.000003463726   ,  \"στN\" -> 0.000003978144   ,  \"τ11 \" -> 0.000000000000   ,  \"τ12\" -> 0.000000000000   ,  \"τ22\" -> 0.000000000000   ,  \"τN1\" -> 0.000000000000   ,  \"τN2\" -> 0.000000000000   ,  \"σηlogτ1 \" -> 0.179978131634   ,  \"σηlogτS\" -> 0.001942969644   ,  \"σηlogτN\" -> 0.143630935441   ,  \"σlogτ1\" -> 0.001593620678   ,  \"σlogτS\" -> 0.000102107372   ,  \"σlogτN\" -> 0.000792653332   ,  \"σητ1\" -> 0.002796559163   ,  \"σητS \" -> 0.000065910181   ,  \"σητN\" -> 0.000720850531    |>   , \r\"IDS0352_210906_RAW_cal__sam_\" ->   <|    \"ζ\" -> 0.036116393265   ,  \"τ1\" -> 0.020310974732   ,  \"τS\" -> 0.044594628397   ,  \"τN\" -> 0.005932938101   ,  \"τC\" -> 0.002747123875   ,  \"κ0\" -> 0.000000002292   ,  \"mm1\" -> 0.000090548575   ,  \"mm2\" -> 0.017024776182   ,  \"mm3\" -> 0.058295213810   ,  \"T\" -> 0.360000000000   ,  \"B\" -> 8.000000000000   ,  \"θ\" -> 90.000000000000   ,  \"Reoff\" -> -2518072.289156645540   ,  \"Imoff\" -> 0.000000000000   ,  \"στ1\" -> 0.000000000000   ,  \"στS\" -> 0.000000000000   ,  \"στN\" -> 0.000000000000   ,  \"τ11 \" -> 0.000000000000   ,  \"τ12\" -> 0.000000000000   ,  \"τ22\" -> 0.000000000000   ,  \"τN1\" -> 0.000000000000   ,  \"τN2\" -> 0.000000000000   ,  \"σηlogτ1 \" -> 0.000000000000   ,  \"σηlogτS\" -> 0.000000000000   ,  \"σηlogτN\" -> 0.000000000000   ,  \"σlogτ1\" -> 0.000000000000   ,  \"σlogτS\" -> 0.000000000000   ,  \"σlogτN\" -> 0.000000000000   ,  \"σητ1\" -> 0.000000000000   ,  \"σητS \" -> 0.000000000000   ,  \"σητN\" -> 0.000000000000    |>   , \r\"IDS0353_210906_RAW_cal__ref_\" ->   <|    \"ζ\" -> 0.043805011586   ,  \"τ1\" -> 0.015641832651   ,  \"τS\" -> 0.031297289619   ,  \"τN\" -> 0.002720036846   ,  \"τC\" -> 0.001830581120   ,  \"κ0\" -> 0.000000002632   ,  \"mm1\" -> 0.000072899501   ,  \"mm2\" -> 0.013753455925   ,  \"mm3\" -> 0.039153514190   ,  \"T\" -> 0.438000000000   ,  \"B\" -> 8.000000000000   ,  \"θ\" -> 90.000000000000   ,  \"Reoff\" -> 0.000000000000   ,  \"Imoff\" -> 0.000000000000   ,  \"στ1\" -> 0.000029789904   ,  \"στS\" -> 0.000002213568   ,  \"στN\" -> 0.000002569992   ,  \"τ11 \" -> 0.000000000000   ,  \"τ12\" -> 0.000000000000   ,  \"τ22\" -> 0.000000000000   ,  \"τN1\" -> 0.000000000000   ,  \"τN2\" -> 0.000000000000   ,  \"σηlogτ1 \" -> 0.171230545078   ,  \"σηlogτS\" -> 0.001043214583   ,  \"σηlogτN\" -> 0.141039696626   ,  \"σlogτ1\" -> 0.001904502144   ,  \"σlogτS\" -> 0.000070727156   ,  \"σlogτN\" -> 0.000944837375   ,  \"σητ1\" -> 0.002678359531   ,  \"σητS \" -> 0.000032649789   ,  \"σητN\" -> 0.000383633172    |>   , \r\"IDS0353_210906_RAW_cal__sam_\" ->   <|    \"ζ\" -> 0.028235631162   ,  \"τ1\" -> 0.018033623612   ,  \"τS\" -> 0.040112967891   ,  \"τN\" -> 0.003332308168   ,  \"τC\" -> 0.002994357278   ,  \"κ0\" -> 0.000000002859   ,  \"mm1\" -> 0.000076791949   ,  \"mm2\" -> 0.016073609718   ,  \"mm3\" -> 0.049549560072   ,  \"T\" -> 0.438000000000   ,  \"B\" -> 8.000000000000   ,  \"θ\" -> 90.000000000000   ,  \"Reoff\" -> -2200000.000000000000   ,  \"Imoff\" -> 0.000000000000   ,  \"στ1\" -> 0.000000000000   ,  \"στS\" -> 0.000000000000   ,  \"στN\" -> 0.000000000000   ,  \"τ11 \" -> 0.000000000000   ,  \"τ12\" -> 0.000000000000   ,  \"τ22\" -> 0.000000000000   ,  \"τN1\" -> 0.000000000000   ,  \"τN2\" -> 0.000000000000   ,  \"σηlogτ1 \" -> 0.000000000000   ,  \"σηlogτS\" -> 0.000000000000   ,  \"σηlogτN\" -> 0.000000000000   ,  \"σlogτ1\" -> 0.000000000000   ,  \"σlogτS\" -> 0.000000000000   ,  \"σlogτN\" -> 0.000000000000   ,  \"σητ1\" -> 0.000000000000   ,  \"σητS \" -> 0.000000000000   ,  \"σητN\" -> 0.000000000000    |>   , \r\"IDS0354_210906_RAW_cal__ref_\" ->   <|    \"ζ\" -> 0.034407438278   ,  \"τ1\" -> 0.012759993552   ,  \"τS\" -> 0.028549472180   ,  \"τN\" -> 0.001373973335   ,  \"τC\" -> 0.002126234468   ,  \"κ0\" -> 0.000000003285   ,  \"mm1\" -> 0.000066111743   ,  \"mm2\" -> 0.011901304001   ,  \"mm3\" -> 0.033871846896   ,  \"T\" -> 0.530000000000   ,  \"B\" -> 8.000000000000   ,  \"θ\" -> 90.000000000000   ,  \"Reoff\" -> 0.000000000000   ,  \"Imoff\" -> 0.000000000000   ,  \"στ1\" -> 0.000105401331   ,  \"στS\" -> 0.000005152140   ,  \"στN\" -> 0.000005607099   ,  \"τ11 \" -> 0.000000000000   ,  \"τ12\" -> 0.000000000000   ,  \"τ22\" -> 0.000000000000   ,  \"τN1\" -> 0.000000000000   ,  \"τN2\" -> 0.000000000000   ,  \"σηlogτ1 \" -> 0.184333164792   ,  \"σηlogτS\" -> 0.000694064017   ,  \"σηlogτN\" -> 0.142381877257   ,  \"σlogτ1\" -> 0.008260296568   ,  \"σlogτS\" -> 0.000180463565   ,  \"σlogτN\" -> 0.004080937594   ,  \"σητ1\" -> 0.002352089994   ,  \"σητS \" -> 0.000019815161   ,  \"σητN\" -> 0.000195628903    |>   , \r\"IDS0354_210906_RAW_cal__sam_\" ->   <|    \"ζ\" -> 0.022962333090   ,  \"τ1\" -> 0.020865157142   ,  \"τS\" -> 0.035948400917   ,  \"τN\" -> 0.001990138096   ,  \"τC\" -> 0.003574397791   ,  \"κ0\" -> 0.000000003542   ,  \"mm1\" -> 0.000073258085   ,  \"mm2\" -> 0.019040364220   ,  \"mm3\" -> 0.044135629011   ,  \"T\" -> 0.530000000000   ,  \"B\" -> 8.000000000000   ,  \"θ\" -> 90.000000000000   ,  \"Reoff\" -> -1700000.000000000000   ,  \"Imoff\" -> 0.000000000000   ,  \"στ1\" -> 0.000000000000   ,  \"στS\" -> 0.000000000000   ,  \"στN\" -> 0.000000000000   ,  \"τ11 \" -> 0.000000000000   ,  \"τ12\" -> 0.000000000000   ,  \"τ22\" -> 0.000000000000   ,  \"τN1\" -> 0.000000000000   ,  \"τN2\" -> 0.000000000000   ,  \"σηlogτ1 \" -> 0.000000000000   ,  \"σηlogτS\" -> 0.000000000000   ,  \"σηlogτN\" -> 0.000000000000   ,  \"σlogτ1\" -> 0.000000000000   ,  \"σlogτS\" -> 0.000000000000   ,  \"σlogτN\" -> 0.000000000000   ,  \"σητ1\" -> 0.000000000000   ,  \"σητS \" -> 0.000000000000   ,  \"σητN\" -> 0.000000000000    |>   , \r\"IDS0355_210906_RAW_cal__ref_\" ->   <|    \"ζ\" -> 0.020775547522   ,  \"τ1\" -> 0.014245155504   ,  \"τS\" -> 0.021871141548   ,  \"τN\" -> 0.000446024292   ,  \"τC\" -> 0.003241636501   ,  \"κ0\" -> 0.000000005421   ,  \"mm1\" -> 0.000057740843   ,  \"mm2\" -> 0.013715964925   ,  \"mm3\" -> 0.026493903416   ,  \"T\" -> 0.830000000000   ,  \"B\" -> 8.000000000000   ,  \"θ\" -> 90.000000000000   ,  \"Reoff\" -> 0.000000000000   ,  \"Imoff\" -> 0.000000000000   ,  \"στ1\" -> 0.000172291727   ,  \"στS\" -> 0.000002161761   ,  \"στN\" -> 0.000002696691   ,  \"τ11 \" -> 0.000000000000   ,  \"τ12\" -> 0.000000000000   ,  \"τ22\" -> 0.000000000000   ,  \"τN1\" -> 0.000000000000   ,  \"τN2\" -> 0.000000000000   ,  \"σηlogτ1 \" -> 0.152304599872   ,  \"σηlogτS\" -> 0.000189712528   ,  \"σηlogτN\" -> 0.136839329472   ,  \"σlogτ1\" -> 0.012094759326   ,  \"σlogτS\" -> 0.000098840802   ,  \"σlogτN\" -> 0.006046063343   ,  \"σητ1\" -> 0.002169602709   ,  \"σητS \" -> 0.000004149230   ,  \"σητN\" -> 0.000061033665    |>   , \r\"IDS0355_210906_RAW_cal__sam_\" ->   <|    \"ζ\" -> 0.015987398390   ,  \"τ1\" -> 0.023974349678   ,  \"τS\" -> 0.025824294014   ,  \"τN\" -> 0.000573136357   ,  \"τC\" -> 0.005688548480   ,  \"κ0\" -> 0.000000005865   ,  \"mm1\" -> 0.000073733721   ,  \"mm2\" -> 0.022561297233   ,  \"mm3\" -> 0.033847323811   ,  \"T\" -> 0.830000000000   ,  \"B\" -> 8.000000000000   ,  \"θ\" -> 90.000000000000   ,  \"Reoff\" -> -599999.999999999999   ,  \"Imoff\" -> 0.000000000000   ,  \"στ1\" -> 0.000000000000   ,  \"στS\" -> 0.000000000000   ,  \"στN\" -> 0.000000000000   ,  \"τ11 \" -> 0.000000000000   ,  \"τ12\" -> 0.000000000000   ,  \"τ22\" -> 0.000000000000   ,  \"τN1\" -> 0.000000000000   ,  \"τN2\" -> 0.000000000000   ,  \"σηlogτ1 \" -> 0.000000000000   ,  \"σηlogτS\" -> 0.000000000000   ,  \"σηlogτN\" -> 0.000000000000   ,  \"σlogτ1\" -> 0.000000000000   ,  \"σlogτS\" -> 0.000000000000   ,  \"σlogτN\" -> 0.000000000000   ,  \"σητ1\" -> 0.000000000000   ,  \"σητS \" -> 0.000000000000   ,  \"σητN\" -> 0.000000000000    |>   , \r\"IDS0359_210907_RAW_cal__ref_\" ->   <|    \"ζ\" -> 0.424845059741   ,  \"τ1\" -> 0.089321051678   ,  \"τS\" -> 0.116595960023   ,  \"τN\" -> 0.612122896867   ,  \"τC\" -> 0.001120095408   ,  \"κ0\" -> 0.000000000383   ,  \"mm1\" -> 0.000332370585   ,  \"mm2\" -> 0.013372321421   ,  \"mm3\" -> 1.115047918259   ,  \"T\" -> 0.120000000000   ,  \"B\" -> 12.000000000000   ,  \"θ\" -> 60.000000000000   ,  \"Reoff\" -> 0.000000000000   ,  \"Imoff\" -> 0.000000000000   ,  \"στ1\" -> 0.000839647107   ,  \"στS\" -> 0.000700328201   ,  \"στN\" -> 0.003352050812   ,  \"τ11 \" -> 0.000000000000   ,  \"τ12\" -> 0.000000000000   ,  \"τ22\" -> 0.000000000000   ,  \"τN1\" -> 0.000000000000   ,  \"τN2\" -> 0.000000000000   ,  \"σηlogτ1 \" -> 0.058996717292   ,  \"σηlogτS\" -> 0.003693056048   ,  \"σηlogτN\" -> 0.066658525220   ,  \"σlogτ1\" -> 0.009400327147   ,  \"σlogτS\" -> 0.006006453401   ,  \"σlogτN\" -> 0.005476107542   ,  \"σητ1\" -> 0.005269648834   ,  \"σητS \" -> 0.000430595415   ,  \"σητN\" -> 0.040803209559    |>   , \r\"IDS0359_210907_RAW_cal__sam_\" ->   <|    \"ζ\" -> 0.241762987309   ,  \"τ1\" -> 0.090301757431   ,  \"τS\" -> 0.104468976957   ,  \"τN\" -> 0.810352557873   ,  \"τC\" -> 0.001702208121   ,  \"κ0\" -> 0.000000000500   ,  \"mm1\" -> 0.000327834342   ,  \"mm2\" -> 0.009723084216   ,  \"mm3\" -> 1.217944568939   ,  \"T\" -> 0.120000000000   ,  \"B\" -> 12.000000000000   ,  \"θ\" -> 60.000000000000   ,  \"Reoff\" -> -52289156.626506023100   ,  \"Imoff\" -> 0.000000000000   ,  \"στ1\" -> 0.000000000000   ,  \"στS\" -> 0.000000000000   ,  \"στN\" -> 0.000000000000   ,  \"τ11 \" -> 0.000000000000   ,  \"τ12\" -> 0.000000000000   ,  \"τ22\" -> 0.000000000000   ,  \"τN1\" -> 0.000000000000   ,  \"τN2\" -> 0.000000000000   ,  \"σηlogτ1 \" -> 0.000000000000   ,  \"σηlogτS\" -> 0.000000000000   ,  \"σηlogτN\" -> 0.000000000000   ,  \"σlogτ1\" -> 0.000000000000   ,  \"σlogτS\" -> 0.000000000000   ,  \"σlogτN\" -> 0.000000000000   ,  \"σητ1\" -> 0.000000000000   ,  \"σητS \" -> 0.000000000000   ,  \"σητN\" -> 0.000000000000    |>   , \r\"IDS0360_210907_RAW_cal__ref_\" ->   <|    \"ζ\" -> 0.342434399581   ,  \"τ1\" -> 0.078890152129   ,  \"τS\" -> 0.062757285209   ,  \"τN\" -> 0.289377193045   ,  \"τC\" -> 0.000956599249   ,  \"κ0\" -> 0.000000000628   ,  \"mm1\" -> 0.000241931953   ,  \"mm2\" -> 0.012416031233   ,  \"mm3\" -> 0.539906225078   ,  \"T\" -> 0.150000000000   ,  \"B\" -> 12.000000000000   ,  \"θ\" -> 60.000000000000   ,  \"Reoff\" -> 0.000000000000   ,  \"Imoff\" -> 0.000000000000   ,  \"στ1\" -> 0.000259479640   ,  \"στS\" -> 0.000106061605   ,  \"στN\" -> 0.000644908503   ,  \"τ11 \" -> 0.000000000000   ,  \"τ12\" -> 0.000000000000   ,  \"τ22\" -> 0.000000000000   ,  \"τN1\" -> 0.000000000000   ,  \"τN2\" -> 0.000000000000   ,  \"σηlogτ1 \" -> 0.046682907310   ,  \"σηlogτS\" -> 0.002342389923   ,  \"σηlogτN\" -> 0.056973626918   ,  \"σlogτ1\" -> 0.003289125866   ,  \"σlogτS\" -> 0.001690028567   ,  \"σlogτN\" -> 0.002228608605   ,  \"σητ1\" -> 0.003682821660   ,  \"σητS \" -> 0.000147002032   ,  \"σητN\" -> 0.016486868235    |>   , \r\"IDS0360_210907_RAW_cal__sam_\" ->   <|    \"ζ\" -> 0.201278537585   ,  \"τ1\" -> 0.081544073952   ,  \"τS\" -> 0.088995303529   ,  \"τN\" -> 0.405130496924   ,  \"τC\" -> 0.001460686320   ,  \"κ0\" -> 0.000000000739   ,  \"mm1\" -> 0.000241947199   ,  \"mm2\" -> 0.013299947862   ,  \"mm3\" -> 0.663045584163   ,  \"T\" -> 0.150000000000   ,  \"B\" -> 12.000000000000   ,  \"θ\" -> 60.000000000000   ,  \"Reoff\" -> -39048192.771084338400   ,  \"Imoff\" -> 0.000000000000   ,  \"στ1\" -> 0.000000000000   ,  \"στS\" -> 0.000000000000   ,  \"στN\" -> 0.000000000000   ,  \"τ11 \" -> 0.000000000000   ,  \"τ12\" -> 0.000000000000   ,  
